vi "rsidr_core_global.vi"() -> ()   [LabVIEW 2020, in "Rohde&Schwarz RTx Oscilloscopes.lvlib"] (continued)
4", "Value 1"=7.0, "Value 2"=0.0, "Command"="MA4"}, {"Name"="Reference Waveform 1", "Value 1"=8.0, "Value 2"=0.0, "Command"="RE1"}, {"Name"="Reference Waveform 2", "Value 1"=9.0, "Value 2"=0.0, "Command"="RE2"}, {"Name"="Reference Waveform 3", "Value 1"=10.0, "Value 2"=0.0, "Command"="RE3"}, {"Name"="Reference Waveform 4", "Value 1"=11.0, "Value 2"=0.0, "Command"="RE4"}, {"Name"="SerialBus 1", "Value 1"=12.0, "Value 2"=0.0, "Command"="SBUS1"}, {"Name"="SerialBus 2", "Value 1"=13.0, "Value 2"=0.0, "Command"="SBUS2"}, {"Name"="SerialBus 3", "Value 1"=14.0, "Value 2"=0.0, "Command"="SBUS3"}, {"Name"="SerialBus 4", "Value 1"=15.0, "Value 2"=0.0, "Command"="SBUS4"}, {"Name"="QMA", "Value 1"=37.0, "Value 2"=0.0, "Command"="QMA"}]}, {"Type"=2, "Name"="rsrtx_rngSearchSlope", "Entries"=[{"Name"="Positive", "Value 1"=0.0, "Value 2"=0.0, "Command"="POS"}, {"Name"="Negative", "Value 1"=1.0, "Value 2"=0.0, "Command"="NEG"}, {"Name"="Either", "Value 1"=2.0, "Value 2"=0.0, "Command"="EITH"}]}, {"Type"=2, "Name"="rsrtx_rngSearchRange", "Entries"=[{"Name"="Shorter", "Value 1"=0.0, "Value 2"=0.0, "Command"="SHOR"}, {"Name"="Longer", "Value 1"=1.0, "Value 2"=0.0, "Command"="LONG"}, {"Name"="Within", "Value 1"=2.0, "Value 2"=0.0, "Command"="WITH"}, {"Name"="Outside", "Value 1"=3.0, "Value 2"=0.0, "Command"="OUTS"}]}, {"Type"=0, "Name"="rsrtx_rngWaveformPosition", "Entries"=[{"Name"="", "Value 1"=-188.0, "Value 2"=212.0, "Command"=""}]}, {"Type"=2, "Name"="rsrtx_rngScalingUnit", "Entries"=[{"Name"="Linear", "Value 1"=0.0, "Value 2"=0.0, "Command"="LIN"}, {"Name"="DBM", "Value 1"=1.0, "Value 2"=0.0, "Command"="DBM"}, {"Name"="DBV", "Value 1"=2.0, "Value 2"=0.0, "Command"="DBV"}]}, {"Type"=2, "Name"="rsrtx_rngProbeUnit", "Entries"=[{"Name"="V", "Value 1"=0.0, "Value 2"=0.0, "Command"="V"}, {"Name"="A", "Value 1"=1.0, "Value 2"=0.0, "Command"="A"}]}, {"Type"=0, "Name"="rsrtx_rngProbeAttenuation", "Entries"=[{"Name"="", "Value 1"=0.0001, "Value 2"=10000.0, "Command"=""}]}, {"Type"=0, "Name"="rsrtx_rngAutoMeasWaveforms", "Entries"=[{"Name"="", "Value 1"=2.0, "Value 2"=1000.0, "Command"=""}]}, {"Type"=2, "Name"="rsrtx_rngWaveformSamplesRange", "Entries"=[{"Name"="Default", "Value 1"=0.0, "Value 2"=0.0, "Command"="DEF"}, {"Name"="Maximum", "Value 1"=1.0, "Value 2"=0.0, "Command"="MAX"}, {"Name"="Display Maximum", "Value 1"=2.0, "Value 2"=0.0, "Command"="DMAX"}]}, {"Type"=2, "Name"="rsrtx_rngMaskTestActionExecution", "Entries"=[{"Name"="Off", "Value 1"=0.0, "Value 2"=0.0, "Command"="OFF"}, {"Name"="Each", "Value 1"=1.0, "Value 2"=0.0, "Command"="EACH"}, {"Name"="Single", "Value 1"=2.0, "Value 2"=0.0, "Command"="SING"}, {"Name"="Cyclic", "Value 1"=3.0, "Value 2"=0.0, "Command"="CYCL"}]}, {"Type"=2, "Name"="rsrtx_rngSearchTriggerPatternCombination", "Entries"=[{"Name"="AND", "Value 1"=0.0, "Value 2"=0.0, "Command"="AND"}, {"Name"="OR", "Value 1"=1.0, "Value 2"=0.0, "Command"="OR"}, {"Name"="NAND", "Value 1"=2.0, "Value 2"=0.0, "Command"="NAND"}, {"Name"="NOR", "Value 1"=3.0, "Value 2"=0.0, "Command"="NOR"}]}, {"Type"=0, "Name"="rsrtx_rngNumberofAverages", "Entries"=[{"Name"="", "Value 1"=2.0, "Value 2"=1024.0, "Command"=""}]}, {"Type"=0, "Name"="rsrtx_rngNumberOfWaveforms", "Entries"=[{"Name"="", "Value 1"=1.0, "Value 2"=10.0, "Command"=""}]}, {"Type"=2, "Name"="rsrtx_rngSearchGateMode", "Entries"=[{"Name"="All", "Value 1"=0.0, "Value 2"=0.0, "Command"="OFF"}, {"Name"="Display", "Value 1"=1.0, "Value 2"=0.0, "Command"="DISP"}, {"Name"="User", "Value 1"=2.0, "Value 2"=0.0, "Command"="ABS"}]}, {"Type"=2, "Name"="rsrtx_rngProtocolSPITriggerSource", "Entries"=[{"Name"="MISO", "Value 1"=3.0, "Value 2"=0.0, "Command"="MISO"}, {"Name"="MOSI", "Value 1"=4.0, "Value 2"=0.0, "Command"="MOSI"}]}, {"Type"=2, "Name"="rsrtx_rngProtocolLINStandard", "Entries"=[{"Name"="Auto", "Value 1"=0.0, "Value 2"=0.0, "Command"="AUTO"}, {"Name"="v 1.x", "Value 1"=1.0, "Value 2"=0.0, "Command"="V1X"}, {"Name"="v 2.x", "Value 1"=2.0, "Value 2"=0.0, "Command"="V2X"}, {"Name"="J2602", "Value 1"=3.0, "Value 2"=0.0, "Command"="J2602"}]}, {"Type"=2, "Name"="rsrtx_rngProtocolLINTriggerMode", "Entries"=[{"Name"="Start", "Value 1"=0.0, "Value 2"=0.0, "Command"="SYNC"}, {"Name"="Identifier", "Value 1"=1.0, "Value 2"=0.0, "Command"="ID"}, {"Name"="Identifier + Data", "Value 1"=2.0, "Value 2"=0.0, "Command"="IDDT"}, {"Name"="Wakeup Frame", "Value 1"=3.0, "Value 2"=0.0, "Command"="WKFR"}, {"Name"="Error Condition", "Value 1"=4.0, "Value 2"=0.0, "Command"="ERRC"}]}, {"Type"=2, "Name"="rsrtx_rngProtocolCondition", "Entries"=[{"Name"="!= Not equal", "Value 1"=0.0, "Value 2"=0.0, "Command"="NEQ"}, {"Name"="=  Equal", "Value 1"=1.0, "Value 2"=0.0, "Command"="EQU"}, {"Name"="<  Less than", "Value 1"=2.0, "Value 2"=0.0, "Command"="LTH"}, {"Name"=">  Greater than", "Value 1"=3.0, "Value 2"=0.0, "Command"="GTH"}]}, {"Type"=0, "Name"="rsrtx_rngProtocolCANDataLength", "Entries"=[{"Name"="", "Value 1"=0.0, "Value 2"=8.0, "Command"=""}]}, {"Type"=2, "Name"="rsrtx_rngProtocolSearchEvent", "Entries"=[{"Name"="Frame", "Value 1"=0.0, "Value 2"=0.0, "Command"="FRAM"}, {"Name"="Error", "Value 1"=1.0, "Value 2"=0.0, "Command"="ERR"}, {"Name"="Identifier", "Value 1"=2.0, "Value 2"=0.0, "Command"="IDEN"}, {"Name"="ID and Data", "Value 1"=3.0, "Value 2"=0.0, "Command"="IDD"}, {"Name"="ID Error", "Value 1"=4.0, "Value 2"=0.0, "Command"="IDER"}]}, {"Type"=2, "Name"="rsrtx_rngProtocolLINSearchFrameSetup", "Entries"=[{"Name"="Start", "Value 1"=0.0, "Value 2"=0.0, "Command"="SOF"}, {"Name"="Wakeup", "Value 1"=1.0, "Value 2"=0.0, "Command"="WAK"}]}, {"Type"=2, "Name"="rsrtx_rngProtocolCANLineType", "Entries"=[{"Name"="CAN-Low", "Value 1"=0.0, "Value 2"=0.0, "Command"="CANL"}, {"Name"="CAN-High", "Value 1"=1.0, "Value 2"=0.0, "Command"="CANH"}]}, {"Type"=0, "Name"="rsrtx_rngProtocolCANBitRate", "Entries"=[{"Name"="", "Value 1"=100.0, "Value 2"=5040000.0, "Command"=""}]}, {"Type"=0, "Name"="rsrtx_rngProtocolCANSamplePoint", "Entries"=[{"Name"="", "Value 1"=10.0, "Value 2"=90.0, "Command"=""}]}, {"Type"=2, "Name"="rsrtx_rngProtocolCANTriggerMode", "Entries"=[{"Name"="Start", "Value 1"=0.0, "Value 2"=0.0, "Command"="STOF"}, {"Name"="End", "Value 1"=1.0, "Value 2"=0.0, "Command"="EOF"}, {"Name"="Identifier", "Value 1"=2.0, "Value 2"=0.0, "Command"="ID"}, {"Name"="Identifier + Data", "Value 1"=3.0, "Value 2"=0.0, "Command"="IDDT"}, {"Name"="Frame Type", "Value 1"=4.0, "Value 2"=0.0, "Command"="FTYP"}, {"Name"="Error Condition", "Value 1"=5.0, "Value 2"=0.0, "Command"="ERRC"}]}, {"Type"=2, "Name"="rsrtx_rngProtocolCANTriggerFrameType", "Entries"=[{"Name"="Data", "Value 1"=0.0, "Value 2"=0.0, "Command"="DATA"}, {"Name"="Remote", "Value 1"=1.0, "Value 2"=0.0, "Command"="REM"}, {"Name"="Error", "Value 1"=2.0, "Value 2"=0.0, "Command"="ERR"}, {"Name"="Over Load", "Value 1"=3.0, "Value 2"=0.0, "Command"="OVER"}, {"Name"="Any", "Value 1"=4.0, "Value 2"=0.0, "Command"="ANY"}]}, {"Type"=2, "Name"="rsrtx_rngProtocolCANIDType", "Entries"=[{"Name"="Standard format", "Value 1"=0.0, "Value 2"=0.0, "Command"="B11"}, {"Name"="Extended format", "Value 1"=1.0, "Value 2"=0.0, "Command"="B29"}, {"Name"="Any", "Value 1"=2.0, "Value 2"=0.0, "Command"="ANY"}]}, {"Type"=2, "Name"="rsrtx_rngProtocolCANSearchFrameSetup", "Entries"=[{"Name"="Start of Frame", "Value 1"=0.0, "Value 2"=0.0, "Command"="SOF"}, {"Name"="End of Frame", "Value 1"=1.0, "Value 2"=0.0, "Command"="EOF"}, {"Name"="Overload Frame", "Value 1"=2.0, "Value 2"=0.0, "Command"="OVER"}, {"Name"="Error Frame", "Value 1"=3.0, "Value 2"=0.0, "Command"="ERR"}, {"Name"="Data11b", "Value 1"=4.0, "Value 2"=0.0, "Command"="DTA11"}, {"Name"="Data29b", "Value 1"=5.0, "Value 2"=0.0, "Command"="DTA29"}, {"Name"="Remote11b", "Value 1"=6.0, "Value 2"=0.0, "Command"="REM11"}, {"Name"="Remote29b", "Value 1"=7.0, "Value 2"=0.0, "Command"="REM29"}]}, {"Type"=2, "Name"="rsrtx_rngProtocolCANSearchFrameType", "Entries"=[{"Name"="Data", "Value 1"=0.0, "Value 2"=0.0, "Command"="DATA"}, {"Name"="Remote", "Value 1"=1.0, "Value 2"=0.0, "Command"="REM"}, {"Name"="Any", "Value 1"=2.0, "Value 2"=0.0, "Command"="ANY"}]}, {"Type"=2, "Name"="rsrtx_rngProtocolLINPolarity", "Entries"=[{"Name"="Low active", "Value 1"=0.0, "Value 2"=0.0, "Command"="IDLH"}, {"Name"="High active", "Value 1"=1.0, "Value 2"=0.0, "Command"="IDLL"}]}, {"Type"=2, "Name"="rsrtx_rngProtocolSPIMISOPolarity", "Entries"=[{"Name"="Low active", "Value 1"=0.0, "Value 2"=0.0, "Command"="ACTL"}, {"Name"="High active", "Value 1"=1.0, "Value 2"=0.0, "Command"="ACTH"}]}, {"Type"=0, "Name"="rsrtx_rngAutomaticMeasurementResultIndex", "Entries"=[{"Name"="", "Value 1"=0.0, "Value 2"=999.0, "Command"=""}]}, {"Type"=2, "Name"="rsrtx_rngDigitalHysteresis", "Entries"=[{"Name"="Small", "Value 1"=0.0, "Value 2"=0.0, "Command"="SMAL"}, {"Name"="Medium", "Value 1"=1.0, "Value 2"=0.0, "Command"="MED"}, {"Name"="Large", "Value 1"=2.0, "Value 2"=0.0, "Command"="LARG"}]}, {"Type"=2, "Name"="rsrtx_rngTriggerHoldoffMode", "Entries"=[{"Name"="Time", "Value 1"=0.0, "Value 2"=0.0, "Command"="TIME"}, {"Name"="Off", "Value 1"=1.0, "Value 2"=0.0, "Command"="OFF"}]}, {"Type"=2, "Name"="rsrtx_rngTriggerPatternMode", "Entries"=[{"Name"="Off", "Value 1"=0.0, "Value 2"=0.0, "Command"="OFF"}, {"Name"="Timeout", "Value 1"=1.0, "Value 2"=0.0, "Command"="TIM"}, {"Name"="Width", "Value 1"=2.0, "Value 2"=0.0, "Command"="WIDT"}]}, {"Type"=2, "Name"="rsrtx_rngTriggerOutMode", "Entries"=[{"Name"="Off", "Value 1"=0.0, "Value 2"=0.0, "Command"="OFF"}, {"Name"="Trigger", "Value 1"=1.0, "Value 2"=0.0, "Command"="TRIG"}, {"Name"="Mask", "Value 1"=2.0, "Value 2"=0.0, "Command"="MASK"}, {"Name"="Reference", "Value 1"=3.0, "Value 2"=0.0, "Command"="REF"}, {"Name"="Generator", "Value 1"=4.0, "Value 2"=0.0, "Command"="GEN"}]}, {"Type"=2, "Name"="rsrtx_rngDigitalTechnology", "Entries"=[{"Name"="TTL", "Value 1"=0.0, "Value 2"=0.0, "Command"="TTL"}, {"Name"="ECL", "Value 1"=1.0, "Value 2"=0.0, "Command"="ECL"}, {"Name"="CMOS", "Value 1"=2.0, "Value 2"=0.0, "Command"="CMOS"}, {"Name"="Manual", "Value 1"=3.0, "Value 2"=0.0, "Command"="MAN"}]}, {"Type"=2, "Name"="rsrtx_rngParallelBusFrameEnabled", "Entries"=[{"Name"="Ok", "Value 1"=0.0, "Value 2"=0.0, "Command"="OK"}, {"Name"="Error", "Value 1"=1.0, "Value 2"=0.0, "Command"="ERR"}, {"Name"="Insufficient", "Value 1"=2.0, "Value 2"=0.0, "Command"="INS"}]}, {"Type"=2, "Name"="rsrtx_rngI2CFrameTransferDirection", "Entries"=[{"Name"="Incomplete", "Value 1"=0.0, "Value 2"=0.0, "Command"="INC"}, {"Name"="Read", "Value 1"=1.0, "Value 2"=0.0, "Command"="READ"}, {"Name"="Write", "Value 1"=2.0, "Value 2"=0.0, "Command"="WRITE"}, {"Name"="Either", "Value 1"=3.0, "Value 2"=0.0, "Command"="EITH"}, {"Name"="Undefined", "Value 1"=4.0, "Value 2"=0.0, "Command"="UNDF"}]}, {"Type"=2, "Name"="rsrtx_rngFrameAddressLength", "Entries"=[{"Name"="7 Bit", "Value 1"=0.0, "Value 2"=0.0, "Command"="BIT7"}, {"Name"="10 Bit", "Value 1"=1.0, "Value 2"=0.0, "Command"="BIT10"}]}, {"Type"=2, "Name"="rsrtx_rngLINFrameStatus", "Entries"=[{"Name"="Ok", "Value 1"=0.0, "Value 2"=0.0, "Command"="OK"}, {"Name"="UART", "Value 1"=1.0, "Value 2"=0.0, "Command"="UART"}, {"Name"="Checksum", "Value 1"=2.0, "Value 2"=0.0, "Command"="CHCK"}, {"Name"="Protocol Error", "Value 1"=3.0, "Value 2"=0.0, "Command"="PRER"}, {"Name"="System Error", "Value 1"=4.0, "Value 2"=0.0, "Command"="SYER"}, {"Name"="Weakup", "Value 1"=5.0, "Value 2"=0.0, "Command"="WAK"}, {"Name"="Insufficient", "Value 1"=6.0, "Value 2"=0.0, "Command"="INS"}, {"Name"="Error", "Value 1"=7.0, "Value 2"=0.0, "Command"="ERR"}, {"Name"="Lener", "Value 1"=8.0, "Value 2"=0.0, "Command"="LEN"}]}, {"Type"=2, "Name"="rsrtx_rngLINChecksum", "Entries"=[{"Name"="Ok", "Value 1"=0.0, "Value 2"=0.0, "Command"="OK"}, {"Name"="Error", "Value 1"=1.0, "Value 2"=0.0, "Command"="ERR"}, {"Name"="Undefined", "Value 1"=2.0, "Value 2"=0.0, "Command"="UNDF"}]}, {"Type"=2, "Name"="rsrtx_rngLINParity", "Entries"=[{"Name"="Ok", "Value 1"=0.0, "Value 2"=0.0, "Command"="OK"}, {"Name"="Parity Error", "Value 1"=1.0, "Value 2"=0.0, "Command"="PRER"}, {"Name"="Unexpected Value", "Value 1"=2.0, "Value 2"=0.0, "Command"="UVAL"}, {"Name"="Insufficient", "Value 1"=3.0, "Value 2"=0.0, "Command"="INS"}]}, {"Type"=2, "Name"="rsrtx_rngLINFrameVersion", "Entries"=[{"Name"="V1X", "Value 1"=0.0, "Value 2"=0.0, "Command"="V1X"}, {"Name"="V2X", "Value 1"=1.0, "Value 2"=0.0, "Command"="V2X"}, {"Name"="Unknown", "Value 1"=2.0, "Value 2"=0.0, "Command"="UNK"}]}, {"Type"=2, "Name"="rsrtx_rngLINByteEnabled", "Entries"=[{"Name"="Ok", "Value 1"=0.0, "Value 2"=0.0, "Command"="OK"}, {"Name"="Insufficient", "Value 1"=1.0, "Value 2"=0.0, "Command"="INS"}, {"Name"="UART", "Value 1"=2.0, "Value 2"=0.0, "Command"="UART"}]}, {"Type"=2, "Name"="rsrtx_rngUARTWordEnabled", "Entries"=[{"Name"="Ok", "Value 1"=0.0, "Value 2"=0.0, "Command"="OK"}, {"Name"="Frst", "Value 1"=1.0, "Value 2"=0.0, "Command"="FRST"}, {"Name"="Fren", "Value 1"=2.0, "Value 2"=0.0, "Command"="FREN"}, {"Name"="Frme", "Value 1"=3.0, "Value 2"=0.0, "Command"="FRME"}, {"Name"="Ster", "Value 1"=4.0, "Value 2"=0.0, "Command"="STER"}, {"Name"="Sper", "Value 1"=5.0, "Value 2"=0.0, "Command"="SPER"}, {"Name"="Prer", "Value 1"=6.0, "Value 2"=0.0, "Command"="PRER"}, {"Name"="Insufficient", "Value 1"=7.0, "Value 2"=0.0, "Command"="INS"}, {"Name"="Break", "Value 1"=8.0, "Value 2"=0.0, "Command"="BRE"}]}, {"Type"=2, "Name"="rsrtx_rngCANFrameType", "Entries"=[{"Name"="Data", "Value 1"=0.0, "Value 2"=0.0, "Command"="DATA"}, {"Name"="Remote", "Value 1"=1.0, "Value 2"=0.0, "Command"="REM"}, {"Name"="Error", "Value 1"=2.0, "Value 2"=0.0, "Command"="ERR"}, {"Name"="Overload", "Value 1"=3.0, "Value 2"=0.0, "Command"="OVLD"}]}, {"Type"=2, "Name"="rsrtx_rngCANFrameStatus", "Entries"=[{"Name"="Ok", "Value 1"=0.0, "Value 2"=0.0, "Command"="OK"}, {"Name"="Bit Stuffing Error", "Value 1"=1.0, "Value 2"=0.0, "Command"="BTST"}, {"Name"="Wrong CRC", "Value 1"=2.0, "Value 2"=0.0, "Command"="CRCD"}, {"Name"="Wrong ACK", "Value 1"=3.0, "Value 2"=0.0, "Command"="ACKD"}, {"Name"="CRC", "Value 1"=4.0, "Value 2"=0.0, "Command"="CRC"}, {"Name"="Wrong End of Frame", "Value 1"=5.0, "Value 2"=0.0, "Command"="EOFD"}, {"Name"="Acknowledge Missing", "Value 1"=6.0, "Value 2"=0.0, "Command"="NOAC"}, {"Name"="Insufficient", "Value 1"=7.0, "Value 2"=0.0, "Command"="INS"}]}, {"Type"=2, "Name"="rsrtx_rngCANAckState", "Entries"=[{"Name"="Ok", "Value 1"=0.0, "Value 2"=0.0, "Command"="OK"}, {"Name"="Undefined", "Value 1"=1.0, "Value 2"=0.0, "Command"="UNDF"}]}, {"Type"=2, "Name"="rsrtx_rngMeasurementSource", "Entries"=[{"Name"="None", "Value 1"=0.0, "Value 2"=0.0, "Command"="NONE"}, {"Name"="Channel 1", "Value 1"=1.0, "Value 2"=0.0, "Command"="CH1"}, {"Name"="Channel 2", "Value 1"=2.0, "Value 2"=0.0, "Command"="CH2"}, {"Name"="Channel 3", "Value 1"=3.0, "Value 2"=0.0, "Command"="CH3"}, {"Name"="Channel 4", "Value 1"=4.0, "Value 2"=0.0, "Command"="CH4"}, {"Name"="Math 1", "Value 1"=5.0, "Value 2"=0.0, "Command"="MA1"}, {"Name"="Math 2", "Value 1"=6.0, "Value 2"=0.0, "Command"="MA2"}, {"Name"="Math 3", "Value 1"=7.0, "Value 2"=0.0, "Command"="MA3"}, {"Name"="Math 4", "Value 1"=8.0, "Value 2"=0.0, "Command"="MA4"}, {"Name"="Math 5", "Value 1"=9.0, "Value 2"=0.0, "Command"="MA5"}, {"Name"="Reference 1", "Value 1"=10.0, "Value 2"=0.0, "Command"="R1"}, {"Name"="Reference 2", "Value 1"=11.0, "Value 2"=0.0, "Command"="R2"}, {"Name"="Reference 3", "Value 1"=12.0, "Value 2"=0.0, "Command"="R3"}, {"Name"="Reference 4", "Value 1"=13.0, "Value 2"=0.0, "Command"="R4"}, {"Name"="Trigger", "Value 1"=14.0, "Value 2"=0.0, "Command"="TRIG"}, {"Name"="Digital Channel 1", "Value 1"=15.0, "Value 2"=0.0, "Command"="D1"}, {"Name"="Digital Channel 2", "Value 1"=16.0, "Value 2"=0.0, "Command"="D2"}, {"Name"="Digital Channel 3", "Value 1"=17.0, "Value 2"=0.0, "Command"="D3"}, {"Name"="Digital Channel 4", "Value 1"=18.0, "Value 2"=0.0, "Command"="D4"}, {"Name"="Digital Channel 5", "Value 1"=19.0, "Value 2"=0.0, "Command"="D5"}, {"Name"="Digital Channel 6", "Value 1"=20.0, "Value 2"=0.0, "Command"="D6"}, {"Name"="Digital Channel 7", "Value 1"=21.0, "Value 2"=0.0, "Command"="D7"}, {"Name"="Digital Channel 8", "Value 1"=22.0, "Value 2"=0.0, "Command"="D8"}, {"Name"="Digital Channel 9", "Value 1"=23.0, "Value 2"=0.0, "Command"="D9"}, {"Name"="Digital Channel 10", "Value 1"=24.0, "Value 2"=0.0, "Command"="D10"}, {"Name"="Digital Channel 11", "Value 1"=25.0, "Value 2"=0.0, "Command"="D11"}, {"Name"="Digital Channel 12", "Value 1"=26.0, "Value 2"=0.0, "Command"="D12"}, {"Name"="Digital Channel 13", "Value 1"=27.0, "Value 2"=0.0, "Command"="D13"}, {"Name"="Digital Channel 14", "Value 1"=28.0, "Value 2"=0.0, "Command"="D14"}, {"Name"="Digital Channel 15", "Value 1"=29.0, "Value 2"=0.0, "Command"="D15"}, {"Name"="D0...D7", "Value 1"=30.0, "Value 2"=0.0, "Command"="D70"}, {"Name"="D8...D15", "Value 1"=31.0, "Value 2"=0.0, "Command"="D158"}, {"Name"="Digital Channel 0", "Value 1"=32.0, "Value 2"=0.0, "Command"="D0"}, {"Name"="Spectrum", "Value 1"=33.0, "Value 2"=0.0, "Command"="SPEC"}, {"Name"="Minimum Hold", "Value 1"=34.0, "Value 2"=0.0, "Command"="MINH"}, {"Name"="Maximum Hold", "Value 1"=35.0, "Value 2"=0.0, "Command"="MAXH"}, {"Name"="Average", "Value 1"=36.0, "Value 2"=0.0, "Command"="AVER"}, {"Name"="QMA", "Value 1"=37.0, "Value 2"=0.0, "Command"="QMA"}]}, {"Type"=2, "Name"="rsrtx_rngPowerAnalysisType", "Entries"=[{"Name"="Off", "Value 1"=0.0, "Value 2"=0.0, "Command"="OFF"}, {"Name"="Quality", "Value 1"=1.0, "Value 2"=0.0, "Command"="QUAL"}, {"Name"="Consumption", "Value 1"=2.0, "Value 2"=0.0, "Command"="CONS"}, {"Name"="Current Harmonics", "Value 1"=3.0, "Value 2"=0.0, "Command"="HARM"}, {"Name"="Ripple", "Value 1"=4.0, "Value 2"=0.0, "Command"="RIPP"}, {"Name"="Spectrum", "Value 1"=5.0, "Value 2"=0.0, "Command"="SPEC"}, {"Name"="Slewrate", "Value 1"=6.0, "Value 2"=0.0, "Command"="SLEW"}, {"Name"="Dynamic On Resistance", "Value 1"=7.0, "Value 2"=0.0, "Command"="DONR"}, {"Name"="Efficiency", "Value 1"=8.0, "Value 2"=0.0, "Command"="EFF"}, {"Name"="Turn Off", "Value 1"=9.0, "Value 2"=0.0, "Command"="TURN"}, {"Name"="Transient", "Value 1"=10.0, "Value 2"=0.0, "Command"="TRAN"}, {"Name"="Switchingloss", "Value 1"=11.0, "Value 2"=0.0, "Command"="SWIT"}, {"Name"="Modulation", "Value 1"=12.0, "Value 2"=0.0, "Command"="MOD"}, {"Name"="Inrush Current", "Value 1"=13.0, "Value 2"=0.0, "Command"="INR"}, {"Name"="Safe Operating Area", "Value 1"=14.0, "Value 2"=0.0, "Command"="SOA"}]}, {"Type"=2, "Name"="rsrtx_rngStatistics", "Entries"=[{"Name"="Actual", "Value 1"=0.0, "Value 2"=0.0, "Command"="ACT"}, {"Name"="Average", "Value 1"=1.0, "Value 2"=0.0, "Command"="AVG"}, {"Name"="Standard Deviation", "Value 1"=2.0, "Value 2"=0.0, "Command"="STDD"}, {"Name"="Minimum", "Value 1"=3.0, "Value 2"=0.0, "Command"="NPE"}, {"Name"="Maximum", "Value 1"=4.0, "Value 2"=0.0, "Command"="PPE"}, {"Name"="Waveform Count", "Value 1"=5.0, "Value 2"=0.0, "Command"="WFMC"}]}, {"Type"=2, "Name"="rsrtx_rngQualityType", "Entries"=[{"Name"="RMS", "Value 1"=0.0, "Value 2"=0.0, "Command"="RMS"}, {"Name"="Frequency", "Value 1"=1.0, "Value 2"=0.0, "Command"="FREQ"}, {"Name"="Crest Factor", "Value 1"=2.0, "Value 2"=0.0, "Command"="CRES"}]}, {"Type"=2, "Name"="rsrtx_rngQualityTypePower", "Entries"=[{"Name"="Real Power", "Value 1"=0.0, "Value 2"=0.0, "Command"="REAL"}, {"Name"="Reactive", "Value 1"=1.0, "Value 2"=0.0, "Command"="REAC"}, {"Name"="Apparent", "Value 1"=2.0, "Value 2"=0.0, "Command"="APP"}, {"Name"="Factor", "Value 1"=3.0, "Value 2"=0.0, "Command"="PFAC"}, {"Name"="Phase", "Value 1"=4.0, "Value 2"=0.0, "Command"="PHAS"}]}, {"Type"=2, "Name"="rsrtx_rngHarmonicsStandard", "Entries"=[{"Name"="ENA", "Value 1"=0.0, "Value 2"=0.0, "Command"="ENA"}, {"Name"="ENB", "Value 1"=1.0, "Value 2"=0.0, "Command"="ENB"}, {"Name"="ENC", "Value 1"=2.0, "Value 2"=0.0, "Command"="ENC"}, {"Name"="END", "Value 1"=3.0, "Value 2"=0.0, "Command"="END"}, {"Name"="MIL", "Value 1"=4.0, "Value 2"=0.0, "Command"="MIL"}, {"Name"="RTC", "Value 1"=5.0, "Value 2"=0.0, "Command"="RTC"}]}, {"Type"=2, "Name"="rsrtx_rngHarmonicsType", "Entries"=[{"Name"="Violent Count", "Value 1"=0.0, "Value 2"=0.0, "Command"="VCO"}, {"Name"="Frequency", "Value 1"=1.0, "Value 2"=0.0, "Command"="FREQ"}, {"Name"="Level", "Value 1"=2.0, "Value 2"=0.0, "Command"="LEV"}, {"Name"="Minimum", "Value 1"=3.0, "Value 2"=0.0, "Command"="MIN"}, {"Name"="Maximum", "Value 1"=4.0, "Value 2"=0.0, "Command"="MAX"}, {"Name"="Mean", "Value 1"=5.0, "Value 2"=0.0, "Command"="MEAN"}, {"Name"="Limit", "Value 1"=6.0, "Value 2"=0.0, "Command"="LEV:LIM"}, {"Name"="Waveform Count", "Value 1"=7.0, "Value 2"=0.0, "Command"="WFMC"}]}, {"Type"=2, "Name"="rsrtx_rngLimitCheck", "Entries"=[{"Name"="Fail", "Value 1"=0.0, "Value 2"=0.0, "Command"="FAIL"}, {"Name"="Pass", "Value 1"=1.0, "Value 2"=0.0, "Command"="PASS"}]}, {"Type"=2, "Name"="rsrtx_rngRippleType", "Entries"=[{"Name"="Frequency", "Value 1"=0.0, "Value 2"=0.0, "Command"="FREQ"}, {"Name"="Peak", "Value 1"=1.0, "Value 2"=0.0, "Command"="PEAK"}, {"Name"="Standard Deviation", "Value 1"=2.0, "Value 2"=0.0, "Command"="STDD"}, {"Name"="Upper Peak", "Value 1"=3.0, "Value 2"=0.0, "Command"="UPE"}, {"Name"="Lower Peak", "Value 1"=4.0, "Value 2"=0.0, "Command"="LPE"}, {"Name"="Mean", "Value 1"=5.0, "Value 2"=0.0, "Command"="MEAN"}, {"Name"="Period", "Value 1"=6.0, "Value 2"=0.0, "Command"="PER"}, {"Name"="Positive Duty Cycle", "Value 1"=7.0, "Value 2"=0.0, "Command"="PDCY"}, {"Name"="Negative Duty Cycle", "Value 1"=8.0, "Value 2"=0.0, "Command"="NDCY"}]}, {"Type"=2, "Name"="rsrtx_rngSpectrumType", "Entries"=[{"Name"="Frequency", "Value 1"=0.0, "Value 2"=0.0, "Command"="FREQ"}, {"Name"="Level", "Value 1"=1.0, "Value 2"=0.0, "Command"="LEV"}, {"Name"="Minimum", "Value 1"=2.0, "Value 2"=0.0, "Command"="MIN"}, {"Name"="Maximum", "Value 1"=3.0, "Value 2"=0.0, "Command"="MAX"}, {"Name"="Average", "Value 1"=4.0, "Value 2"=0.0, "Command"="MEAN"}, {"Name"="Waveform Count", "Value 1"=5.0, "Value 2"=0.0, "Command"="WFMC"}]}, {"Type"=2, "Name"="rsrtx_rngHarmonicsFundamental", "Entries"=[{"Name"="Auto", "Value 1"=0.0, "Value 2"=0.0, "Command"="AUTO"}, {"Name"="F50", "Value 1"=1.0, "Value 2"=0.0, "Command"="F50"}, {"Name"="F60", "Value 1"=2.0, "Value 2"=0.0, "Command"="F60"}]}, {"Type"=2, "Name"="rsrtx_rngSlewRateType", "Entries"=[{"Name"="Lower Peak", "Value 1"=0.0, "Value 2"=0.0, "Command"="LPE"}, {"Name"="Upper Peak", "Value 1"=1.0, "Value 2"=0.0, "Command"="UPE"}]}, {"Type"=2, "Name"="rsrtx_rngModulationType", "Entries"=[{"Name"="Period", "Value 1"=0.0, "Value 2"=0.0, "Command"="PER"}, {"Name"="Frequency", "Value 1"=1.0, "Value 2"=0.0, "Command"="FREQ"}, {"Name"="Positive Duty Cycle", "Value 1"=2.0, "Value 2"=0.0, "Command"="PDCY"}, {"Name"="Negative Duty Cycle", "Value 1"=3.0, "Value 2"=0.0, "Command"="NDCY"}, {"Name"="Positive Pulse Width", "Value 1"=4.0, "Value 2"=0.0, "Command"="PPW"}, {"Name"="Negative Pulse Width", "Value 1"=5.0, "Value 2"=0.0, "Command"="NPW"}]}, {"Type"=2, "Name"="rsrtx_rngModulationResultType", "Entries"=[{"Name"="Lower Peak", "Value 1"=0.0, "Value 2"=0.0, "Command"="LPE"}, {"Name"="Upper Peak", "Value 1"=1.0, "Value 2"=0.0, "Command"="UPE"}, {"Name"="Mean", "Value 1"=2.0, "Value 2"=0.0, "Command"="MEAN"}, {"Name"="RMS", "Value 1"=3.0, "Value 2"=0.0, "Command"="RMS"}, {"Name"="Standard Deviation", "Value 1"=4.0, "Value 2"=0.0, "Command"="STDD"}]}, {"Type"=2, "Name"="rsrtx_rngEfficiencyType", "Entries"=[{"Name"="Efficiency", "Value 1"=0.0, "Value 2"=0.0, "Command"="EFF"}, {"Name"="Input", "Value 1"=1.0, "Value 2"=0.0, "Command"="INP:REAL"}, {"Name"="Output", "Value 1"=2.0, "Value 2"=0.0, "Command"="OUTP:REAL"}]}, {"Type"=2, "Name"="rsrtx_rngSwitchinglossType", "Entries"=[{"Name"="Energy", "Value 1"=0.0, "Value 2"=0.0, "Command"="ENER"}, {"Name"="Power", "Value 1"=1.0, "Value 2"=0.0, "Command"="POW"}]}, {"Type"=2, "Name"="rsrtx_rngOnOffType", "Entries"=[{"Name"="On", "Value 1"=1.0, "Value 2"=0.0, "Command"="TON"}, {"Name"="Off", "Value 1"=0.0, "Value 2"=0.0, "Command"="TOFF"}]}, {"Type"=2, "Name"="rsrtx_rngPowerAnalysisSource", "Entries"=[{"Name"="Channel 1", "Value 1"=1.0, "Value 2"=0.0, "Command"="CH1"}, {"Name"="Channel 2", "Value 1"=2.0, "Value 2"=0.0, "Command"="CH2"}, {"Name"="Channel 3", "Value 1"=3.0, "Value 2"=0.0, "Command"="CH3"}, {"Name"="Channel 4", "Value 1"=4.0, "Value 2"=0.0, "Command"="CH4"}, {"Name"="RE1", "Value 1"=5.0, "Value 2"=0.0, "Command"="RE1"}, {"Name"="RE2", "Value 1"=6.0, "Value 2"=0.0, "Command"="RE2"}, {"Name"="RE3", "Value 1"=7.0, "Value 2"=0.0, "Command"="RE3"}, {"Name"="RE4", "Value 1"=8.0, "Value 2"=0.0, "Command"="RE4"}]}, {"Type"=2, "Name"="rsrtx_rngAudioVariant", "Entries"=[{"Name"="Inter-IC Sound", "Value 1"=0.0, "Value 2"=0.0, "Command"="I2S"}, {"Name"="Left-justified", "Value 1"=1.0, "Value 2"=0.0, "Command"="LJ"}, {"Name"="Right-justified", "Value 1"=2.0, "Value 2"=0.0, "Command"="RJ"}, {"Name"="Time Division Multiplexed", "Value 1"=3.0, "Value 2"=0.0, "Command"="TDM"}]}, {"Type"=2, "Name"="rsrtx_rngAudioClockPolarity", "Entries"=[{"Name"="Falling", "Value 1"=0.0, "Value 2"=0.0, "Command"="FALL"}, {"Name"="Rising", "Value 1"=1.0, "Value 2"=0.0, "Command"="RIS"}]}, {"Type"=2, "Name"="rsrtx_rngAudioWSPolarity", "Entries"=[{"Name"="Normal", "Value 1"=0.0, "Value 2"=0.0, "Command"="NORM"}, {"Name"="Invert", "Value 1"=1.0, "Value 2"=0.0, "Command"="INV"}]}, {"Type"=2, "Name"="rsrtx_rngAudioChannelOrder", "Entries"=[{"Name"="Left First", "Value 1"=0.0, "Value 2"=0.0, "Command"="LFIR"}, {"Name"="Right First", "Value 1"=1.0, "Value 2"=0.0, "Command"="RFIR"}]}, {"Type"=2, "Name"="rsrtx_rngProtocolAudioBitOrder", "Entries"=[{"Name"="Most significant bit", "Value 1"=0.0, "Value 2"=0.0, "Command"="MSBF"}, {"Name"="Least significant bit", "Value 1"=1.0, "Value 2"=0.0, "Command"="LSBF"}]}, {"Type"=0, "Name"="rsrtx_rngAudioOffset", "Entries"=[{"Name"="", "Value 1"=0.0, "Value 2"=31.0, "Command"=""}]}, {"Type"=0, "Name"="rsrtx_rngAudioTDMChannels", "Entries"=[{"Name"="", "Value 1"=1.0, "Value 2"=8.0, "Command"=""}]}, {"Type"=2, "Name"="rsrtx_rngAudioTriggerType", "Entries"=[{"Name"="Data", "Value 1"=0.0, "Value 2"=0.0, "Command"="DATA"}, {"Name"="Window", "Value 1"=1.0, "Value 2"=0.0, "Command"="WIND"}, {"Name"="Word Select", "Value 1"=2.0, "Value 2"=0.0, "Command"="WSEL"}, {"Name"="Error Condition", "Value 1"=3.0, "Value 2"=0.0, "Command"="ERRC"}]}, {"Type"=0, "Name"="rsrtx_rngProtocolAudioWindowLength", "Entries"=[{"Name"="", "Value 1"=1.0, "Value 2"=1000000.0, "Command"=""}]}, {"Type"=2, "Name"="rsrtx_rngAudioFrameStatus", "Entries"=[{"Name"="OK", "Value 1"=0.0, "Value 2"=0.0, "Command"="OK"}, {"Name"="Error", "Value 1"=1.0, "Value 2"=0.0, "Command"="ERR"}, {"Name"="Insufficient", "Value 1"=2.0, "Value 2"=0.0, "Command"="INS"}]}, {"Type"=0, "Name"="rsrtx_rngAudioFrameOffset", "Entries"=[{"Name"="", "Value 1"=0.0, "Value 2"=31.0, "Command"=""}]}, {"Type"=2, "Name"="rsrtx_rngTrackDisplayMode", "Entries"=[{"Name"="Sequential", "Value 1"=0.0, "Value 2"=0.0, "Command"="SEQ"}, {"Name"="Parallel", "Value 1"=1.0, "Value 2"=0.0, "Command"="PAR"}, {"Name"="Sequential + Track", "Value 1"=2.0, "Value 2"=0.0, "Command"="STR"}, {"Name"="Parallel + Track", "Value 1"=3.0, "Value 2"=0.0, "Command"="PTR"}, {"Name"="Track", "Value 1"=4.0, "Value 2"=0.0, "Command"="TRAC"}, {"Name"="Sequential + Bits", "Value 1"=5.0, "Value 2"=0.0, "Command"="SDS"}]}, {"Type"=2, "Name"="rsrtx_rngAudioTriggerCondition", "Entries"=[{"Name"="Off", "Value 1"=0.0, "Value 2"=0.0, "Command"="OFF"}, {"Name"="Equal", "Value 1"=1.0, "Value 2"=0.0, "Command"="EQU"}, {"Name"="Not Equal", "Value 1"=2.0, "Value 2"=0.0, "Command"="NEQ"}, {"Name"="Greater Than", "Value 1"=3.0, "Value 2"=0.0, "Command"="GTH"}, {"Name"="Less Than", "Value 1"=4.0, "Value 2"=0.0, "Command"="LTH"}, {"Name"="In Range", "Value 1"=5.0, "Value 2"=0.0, "Command"="INR"}, {"Name"="Out Of Range", "Value 1"=6.0, "Value 2"=0.0, "Command"="OOR"}]}, {"Type"=2, "Name"="rsrtx_rngAudioTriggerCombination", "Entries"=[{"Name"="And", "Value 1"=0.0, "Value 2"=0.0, "Command"="AND"}, {"Name"="Or", "Value 1"=1.0, "Value 2"=0.0, "Command"="OR"}]}, {"Type"=2, "Name"="rsrtx_rngSelfAlignmentState", "Entries"=[{"Name"="No Alignment", "Value 1"=0.0, "Value 2"=0.0, "Command"="NOAL"}, {"Name"="Run", "Value 1"=1.0, "Value 2"=0.0, "Command"="RUN"}, {"Name"="Error", "Value 1"=2.0, "Value 2"=0.0, "Command"="ERR"}, {"Name"="Ok", "Value 1"=3.0, "Value 2"=0.0, "Command"="OK"}, {"Name"="Abort", "Value 1"=4.0, "Value 2"=0.0, "Command"="ABOR"}]}, {"Type"=2, "Name"="rsrtx_rngMILSTDCodeType", "Entries"=[{"Name"="Dynamic bus control", "Value 1"=0.0, "Value 2"=0.0, "Command"="DBC"}, {"Name"="Synchronize without data", "Value 1"=1.0, "Value 2"=0.0, "Command"="TSYN"}, {"Name"="Transmit status word", "Value 1"=2.0, "Value 2"=0.0, "Command"="TST"}, {"Name"="Selftest", "Value 1"=3.0, "Value 2"=0.0, "Command"="ISEL"}, {"Name"="Transmitter shutdown", "Value 1"=4.0, "Value 2"=0.0, "Command"="TSH"}, {"Name"="Override transmitter shutdown", "Value 1"=5.0, "Value 2"=0.0, "Command"="OTSH"}, {"Name"="Inhibit terminal flag", "Value 1"=6.0, "Value 2"=0.0, "Command"="ITER"}, {"Name"="Override inhibit terminal flag", "Value 1"=7.0, "Value 2"=0.0, "Command"="OIT"}, {"Name"="Reset remote terminal", "Value 1"=8.0, "Value 2"=0.0, "Command"="RES"}, {"Name"="Transmit vector word", "Value 1"=9.0, "Value 2"=0.0, "Command"="VECT"}, {"Name"="Synchronize with data", "Value 1"=10.0, "Value 2"=0.0, "Command"="RSYN"}, {"Name"="Transmit last command word", "Value 1"=11.0, "Value 2"=0.0, "Command"="TLAS"}, {"Name"="BitWord", "Value 1"=12.0, "Value 2"=0.0, "Command"="BITW"}, {"Name"="Sselected transmitter shutdown", "Value 1"=13.0, "Value 2"=0.0, "Command"="STSH"}, {"Name"="Override selected transmitter shutdown", "Value 1"=14.0, "Value 2"=0.0, "Command"="OSTS"}, {"Name"="Any", "Value 1"=15.0, "Value 2"=0.0, "Command"="ANY"}]}, {"Type"=2, "Name"="rsrtx_rngMILSTDStatus", "Entries"=[{"Name"="Ok", "Value 1"=0.0, "Value 2"=0.0, "Command"="OK"}, {"Name"="Insufficient", "Value 1"=1.0, "Value 2"=0.0, "Command"="INS"}, {"Name"="PError", "Value 1"=2.0, "Value 2"=0.0, "Command"="PERR"}, {"Name"="Message Error", "Value 1"=3.0, "Value 2"=0.0, "Command"="MERR"}, {"Name"="Terror", "Value 1"=4.0, "Value 2"=0.0, "Command"="TERR"}, {"Name"="Serror", "Value 1"=5.0, "Value 2"=0.0, "Command"="SERR"}]}, {"Type"=2, "Name"="rsrtx_rngMILSTDDirection", "Entries"=[{"Name"="Transmit", "Value 1"=0.0, "Value 2"=0.0, "Command"="TRAN"}, {"Name"="Receive", "Value 1"=1.0, "Value 2"=0.0, "Command"="REC"}, {"Name"="Either", "Value 1"=2.0, "Value 2"=0.0, "Command"="EITH"}]}, {"Type"=2, "Name"="rsrtx_rngMILSTDType", "Entries"=[{"Name"="Command", "Value 1"=0.0, "Value 2"=0.0, "Command"="COMM"}, {"Name"="Status", "Value 1"=1.0, "Value 2"=0.0, "Command"="STAT"}, {"Name"="Data", "Value 1"=2.0, "Value 2"=0.0, "Command"="DATA"}, {"Name"="CMCMode", "Value 1"=3.0, "Value 2"=0.0, "Command"="CMCM"}]}, {"Type"=2, "Name"="rsrtx_rngMILSTDTriggerType", "Entries"=[{"Name"="Synchronization", "Value 1"=0.0, "Value 2"=0.0, "Command"="SYNC"}, {"Name"="Frame", "Value 1"=1.0, "Value 2"=0.0, "Command"="FRAM"}, {"Name"="Error", "Value 1"=2.0, "Value 2"=0.0, "Command"="ERR"}, {"Name"="Status", "Value 1"=3.0, "Value 2"=0.0, "Command"="STAT"}, {"Name"="Data", "Value 1"=4.0, "Value 2"=0.0, "Command"="DATA"}, {"Name"="Command", "Value 1"=5.0, "Value 2"=0.0, "Command"="COMM"}, {"Name"="CData", "Value 1"=6.0, "Value 2"=0.0, "Command"="CDAT"}]}, {"Type"=2, "Name"="rsrtx_rngMILSTDTriggerSync", "Entries"=[{"Name"="C/S", "Value 1"=0.0, "Value 2"=0.0, "Command"="CST"}, {"Name"="Data", "Value 1"=1.0, "Value 2"=0.0, "Command"="DATA"}, {"Name"="All", "Value 1"=2.0, "Value 2"=0.0, "Command"="EITH"}]}, {"Type"=2, "Name"="rsrtx_rngMILSTDTriggerWord", "Entries"=[{"Name"="Command", "Value 1"=0.0, "Value 2"=0.0, "Command"="COMM"}, {"Name"="Status", "Value 1"=1.0, "Value 2"=0.0, "Command"="STAT"}, {"Name"="Data", "Value 1"=2.0, "Value 2"=0.0, "Command"="DATA"}, {"Name"="All", "Value 1"=3.0, "Value 2"=0.0, "Command"="ALL"}]}, {"Type"=2, "Name"="rsrtx_rngMILSTDTriggerCommandType", "Entries"=[{"Name"="Triggers on an address or word count", "Value 1"=0.0, "Value 2"=0.0, "Command"="AWOR"}, {"Name"="Triggers on a mode code", "Value 1"=1.0, "Value 2"=0.0, "Command"="MCOD"}]}, {"Type"=2, "Name"="rsrtx_rngMILSTDCondition", "Entries"=[{"Name"="Off", "Value 1"=0.0, "Value 2"=0.0, "Command"="OFF"}, {"Name"="= Equal", "Value 1"=1.0, "Value 2"=0.0, "Command"="EQU"}, {"Name"="!= Not equal", "Value 1"=2.0, "Value 2"=0.0, "Command"="NEQ"}, {"Name"="> Greather Than", "Value 1"=3.0, "Value 2"=0.0, "Command"="GTH"}, {"Name"="=> Greater Equal", "Value 1"=4.0, "Value 2"=0.0, "Command"="GEQ"}, {"Name"="<= Less Equal", "Value 1"=5.0, "Value 2"=0.0, "Command"="LEQ"}, {"Name"="< Less Than", "Value 1"=6.0, "Value 2"=0.0, "Command"="LTH"}, {"Name"="Within", "Value 1"=7.0, "Value 2"=0.0, "Command"="WITH"}, {"Name"="Outside", "Value 1"=8.0, "Value 2"=0.0, "Command"="OUTS"}]}, {"Type"=2, "Name"="rsrtx_rngMILSTDSubAddress", "Entries"=[{"Name"="A0", "Value 1"=0.0, "Value 2"=0.0, "Command"="A0"}, {"Name"="A31", "Value 1"=1.0, "Value 2"=0.0, "Command"="A31"}, {"Name"="Either", "Value 1"=2.0, "Value 2"=0.0, "Command"="EITH"}]}, {"Type"=2, "Name"="rsrtx_rngMILSTDSearchCondition", "Entries"=[{"Name"="Word Start", "Value 1"=0.0, "Value 2"=0.0, "Command"="WST"}, {"Name"="Error", "Value 1"=1.0, "Value 2"=0.0, "Command"="ERR"}, {"Name"="Status", "Value 1"=2.0, "Value 2"=0.0, "Command"="STAT"}, {"Name"="Data", "Value 1"=3.0, "Value 2"=0.0, "Command"="DATA"}, {"Name"="Command", "Value 1"=4.0, "Value 2"=0.0, "Command"="COMM"}, {"Name"="Mode Code", "Value 1"=5.0, "Value 2"=0.0, "Command"="MCOD"}, {"Name"="Command Data", "Value 1"=6.0, "Value 2"=0.0, "Command"="CDAT"}]}, {"Type"=2, "Name"="rsrtx_rngMILSTDSearchError", "Entries"=[{"Name"="Synchronization", "Value 1"=0.0, "Value 2"=0.0, "Command"="SYNC"}, {"Name"="Parity", "Value 1"=1.0, "Value 2"=0.0, "Command"="PAR"}, {"Name"="Timeout", "Value 1"=2.0, "Value 2"=0.0, "Command"="TIM"}, {"Name"="Manchester", "Value 1"=3.0, "Value 2"=0.0, "Command"="MANC"}, {"Name"="Any", "Value 1"=4.0, "Value 2"=0.0, "Command"="ANY"}]}, {"Type"=2, "Name"="rsrtx_rngHistoryPlayer", "Entries"=[{"Name"="Run", "Value 1"=1.0, "Value 2"=0.0, "Command"="RUN"}, {"Name"="Stop", "Value 1"=0.0, "Value 2"=0.0, "Command"="STOP"}]}, {"Type"=2, "Name"="rsrtx_rngHistorySpeed", "Entries"=[{"Name"="Slow", "Value 1"=0.0, "Value 2"=0.0, "Command"="SLOW"}, {"Name"="Medium", "Value 1"=1.0, "Value 2"=0.0, "Command"="MED"}, {"Name"="Fast", "Value 1"=2.0, "Value 2"=0.0, "Command"="FAST"}, {"Name"="Auto", "Value 1"=3.0, "Value 2"=0.0, "Command"="AUTO"}]}, {"Type"=2, "Name"="rsrtx_rngThresholdHysteresis", "Entries"=[{"Name"="Small", "Value 1"=0.0, "Value 2"=0.0, "Command"="SMAL"}, {"Name"="Medium", "Value 1"=1.0, "Value 2"=0.0, "Command"="MED"}, {"Name"="Large", "Value 1"=2.0, "Value 2"=0.0, "Command"="LARG"}]}, {"Type"=2, "Name"="rsrtx_rngStatus", "Entries"=[{"Name"="0", "Value 1"=0.0, "Value 2"=0.0, "Command"="0"}, {"Name"="1", "Value 1"=1.0, "Value 2"=0.0, "Command"="1"}, {"Name"="X", "Value 1"=2.0, "Value 2"=0.0, "Command"="X"}]}, {"Type"=2, "Name"="rsrtx_rngProtocolARINC429Polarity", "Entries"=[{"Name"="A Leg", "Value 1"=0.0, "Value 2"=0.0, "Command"="ALEG"}, {"Name"="B Leg", "Value 1"=1.0, "Value 2"=0.0, "Command"="BLEG"}, {"Name"="Normal", "Value 1"=2.0, "Value 2"=0.0, "Command"="NORM"}, {"Name"="Inverted", "Value 1"=3.0, "Value 2"=0.0, "Command"="INV"}]}, {"Type"=2, "Name"="rsrtx_rngProtocolARINC429BitRateMode", "Entries"=[{"Name"="Low", "Value 1"=0.0, "Value 2"=0.0, "Command"="LOW"}, {"Name"="High", "Value 1"=1.0, "Value 2"=0.0, "Command"="HIGH"}, {"Name"="User", "Value 1"=2.0, "Value 2"=0.0, "Command"="USER"}]}, {"Type"=0, "Name"="rsrtx_rngProtocolARINC429ThresholdHigh", "Entries"=[{"Name"="", "Value 1"=-0.5, "Value 2"=12.0, "Command"=""}]}, {"Type"=0, "Name"="rsrtx_rngProtocolARINC429ThresholdLow", "Entries"=[{"Name"="", "Value 1"=-100.0, "Value 2"=100.0, "Command"=""}]}, {"Type"=2, "Name"="rsrtx_rngARINC429WordStatus", "Entries"=[{"Name"="OK", "Value 1"=0.0, "Value 2"=0.0, "Command"="OK"}, {"Name"="Coding error", "Value 1"=1.0, "Value 2"=0.0, "Command"="CODE"}, {"Name"="Timing gap error", "Value 1"=2.0, "Value 2"=0.0, "Command"="GAP"}, {"Name"="Parity error", "Value 1"=3.0, "Value 2"=0.0, "Command"="PAR"}, {"Name"="Insufficient", "Value 1"=4.0, "Value 2"=0.0, "Command"="INS"}, {"Name"="Incomplete", "Value 1"=5.0, "Value 2"=0.0, "Command"="INC"}]}, {"Type"=2, "Name"="rsrtx_rngProtocolARINC429DataFormat", "Entries"=[{"Name"="Data", "Value 1"=0.0, "Value 2"=0.0, "Command"="DATA"}, {"Name"="SSM+Data", "Value 1"=1.0, "Value 2"=0.0, "Command"="DSSM"}, {"Name"="SDI+Data", "Value 1"=2.0, "Value 2"=0.0, "Command"="DSDI"}, {"Name"="SSM+Data +SDI", "Value 1"=3.0, "Value 2"=0.0, "Command"="DSSS"}]}, {"Type"=2, "Name"="rsrtx_rngProtocolARINC429Operator", "Entries"=[{"Name"="Not equal", "Value 1"=0.0, "Value 2"=0.0, "Command"="NEQ"}, {"Name"="Equal", "Value 1"=1.0, "Value 2"=0.0, "Command"="EQU"}, {"Name"="Less than", "Value 1"=2.0, "Value 2"=0.0, "Command"="LTH"}, {"Name"="Less or equal than", "Value 1"=3.0, "Value 2"=0.0, "Command"="LEQ"}, {"Name"="Greater than", "Value 1"=4.0, "Value 2"=0.0, "Command"="GTH"}, {"Name"="Greater or equal than", "Value 1"=5.0, "Value 2"=0.0, "Command"="GEQ"}, {"Name"="Within", "Value 1"=6.0, "Value 2"=0.0, "Command"="WITH"}, {"Name"="Outside", "Value 1"=7.0, "Value 2"=0.0, "Command"="OUTS"}]}, {"Type"=2, "Name"="rsrtx_rngARINCSsmSdi", "Entries"=[{"Name"="ANY", "Value 1"=0.0, "Value 2"=0.0, "Command"="ANY"}, {"Name"="S00", "Value 1"=1.0, "Value 2"=0.0, "Command"="S00"}, {"Name"="S01", "Value 1"=2.0, "Value 2"=0.0, "Command"="S01"}, {"Name"="S10", "Value 1"=3.0, "Value 2"=0.0, "Command"="S10"}, {"Name"="S11", "Value 1"=4.0, "Value 2"=0.0, "Command"="S11"}]}, {"Type"=2, "Name"="rsrtx_rngARINC429TimingCondition", "Entries"=[{"Name"="Greater than", "Value 1"=0.0, "Value 2"=0.0, "Command"="GTH"}, {"Name"="Less than", "Value 1"=1.0, "Value 2"=0.0, "Command"="LTH"}, {"Name"="Within", "Value 1"=2.0, "Value 2"=0.0, "Command"="WITH"}, {"Name"="Outside", "Value 1"=3.0, "Value 2"=0.0, "Command"="OUTS"}]}, {"Type"=2, "Name"="rsrtx_rngARINC429WordType", "Entries"=[{"Name"="Start", "Value 1"=0.0, "Value 2"=0.0, "Command"="STAR"}, {"Name"="Stop", "Value 1"=1.0, "Value 2"=0.0, "Command"="STOP"}]}, {"Type"=2, "Name"="rsrtx_rngARINC429Type", "Entries"=[{"Name"="Word", "Value 1"=0.0, "Value 2"=0.0, "Command"="WORD"}, {"Name"="Error", "Value 1"=1.0, "Value 2"=0.0, "Command"="ERR"}, {"Name"="Label", "Value 1"=2.0, "Value 2"=0.0, "Command"="LAB"}, {"Name"="Label Data", "Value 1"=3.0, "Value 2"=0.0, "Command"="LDAT"}, {"Name"="Time", "Value 1"=4.0, "Value 2"=0.0, "Command"="TTIM"}]}, {"Type"=2, "Name"="rsrtx_rngARINC429Error", "Entries"=[{"Name"="Any", "Value 1"=0.0, "Value 2"=0.0, "Command"="ANY"}, {"Name"="Parity", "Value 1"=1.0, "Value 2"=0.0, "Command"="PAR"}, {"Name"="Gap", "Value 1"=2.0, "Value 2"=0.0, "Command"="GAP"}, {"Name"="Coding", "Value 1"=3.0, "Value 2"=0.0, "Command"="COD"}]}, {"Type"=2, "Name"="rsrtx_rngMILSTDTransmissionType", "Entries"=[{"Name"="Controller to terminal", "Value 1"=0.0, "Value 2"=0.0, "Command"="BCRT"}, {"Name"="Terminal to controller", "Value 1"=1.0, "Value 2"=0.0, "Command"="RTBC"}, {"Name"="Terminal to terminal", "Value 1"=2.0, "Value 2"=0.0, "Command"="RTRT"}, {"Name"="Mode code data", "Value 1"=3.0, "Value 2"=0.0, "Command"="MCD"}]}, {"Type"=2, "Name"="rsrtx_rngMILSTDSearchWordStart", "Entries"=[{"Name"="Status", "Value 1"=0.0, "Value 2"=0.0, "Command"="STAT"}, {"Name"="Data", "Value 1"=1.0, "Value 2"=0.0, "Command"="DATA"}, {"Name"="Command", "Value 1"=2.0, "Value 2"=0.0, "Command"="COMM"}]}, {"Type"=2, "Name"="rsrtx_rngHardcopyCommandSet", "Entries"=[{"Name"="PCL5", "Value 1"=0.0, "Value 2"=0.0, "Command"="PCL5"}, {"Name"="PCL XI", "Value 1"=1.0, "Value 2"=0.0, "Command"="PCLX"}, {"Name"="Postscript", "Value 1"=2.0, "Value 2"=0.0, "Command"="PS"}, {"Name"="Deskjet", "Value 1"=3.0, "Value 
